vi "Read.ProcessData.ChangeIndexes.vi"(4 "length":i32=-1, 6 "index":i32, 8 "error in (no error)":errorcluster, 10 "timeout ms":i32, 11 "Read in":refnum<class "Read.lvclass">) -> (0 "error out":errorcluster, 1 "Timeout?":bool, 2 "Data":dbl[](array[numeric]), 3 "Read out":refnum<class "Read.lvclass">, 5 "change idexes":i32[](array[numeric]))   [LabVIEW 2015, in "Data Access Engine.lvlib" / "Read.lvclass"]
uses:
  Read.lvclass
  Read.lvclass/Read.ctl
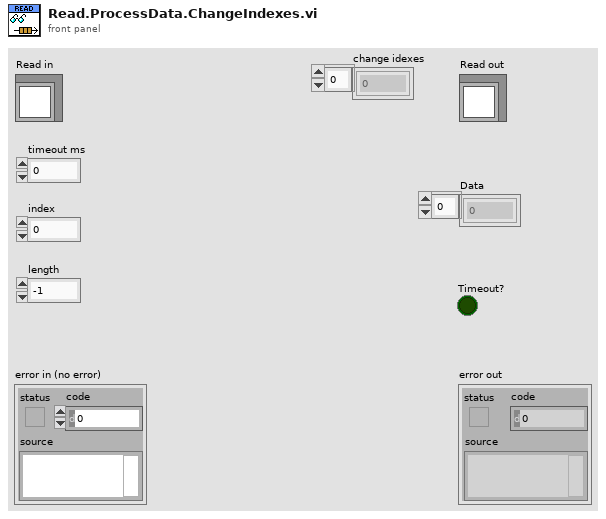
[diagram p1: front panel]
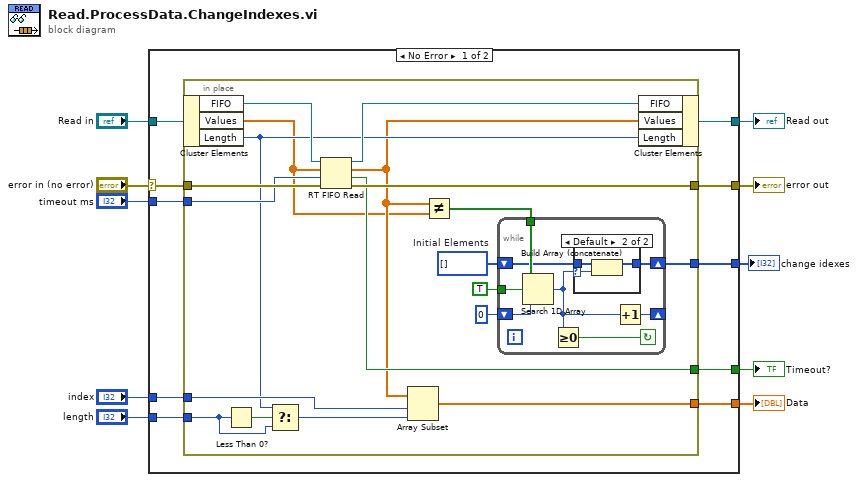
[diagram p0: block diagram]
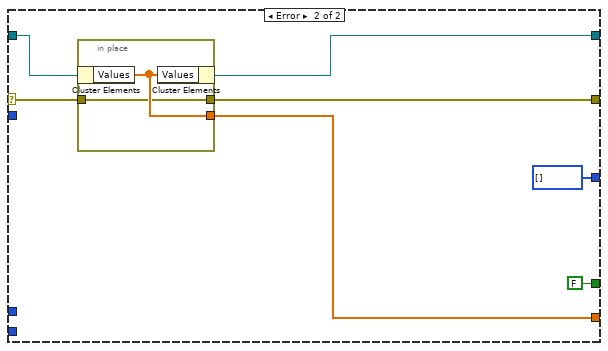
[diagram p3: hidden frame]
diagram:
  n1 = case shown="No Error" "error in (no error)" {
    selector: "error in (no error)" -> [w18 w57]
    tunnel: [w17 w53] -> w9
    tunnel: [w19 w55] -> w7
    tunnel: "Read in" -> [w20 w56]
    tunnel: "timeout ms" -> [w16 _]
    tunnel: [w15 w54] -> w5
    tunnel: [w14 FALSE ("empty?")] -> w4
    tunnel: "length" -> [w13 _]
    tunnel: "index" -> [w12 _]
    tunnel: [w11 i32[] [] ("Initial Elements")] -> w1
    frame No Error {
      n2 = in-place {
        in-place-border: w18 -> [w37]
        in-place-border: [w36] -> w17
        in-place-border: w16 -> [w35]
        in-place-border: [w29] -> w15
        in-place-border: [w34] -> w14
        in-place-border: w13 -> [w32]
        in-place-border: w12 -> [w30]
        in-place-border: [w21] -> w11
        w26 = i32[] []  # Initial Elements
        n3 = in-place-cluster #1(w20) -> ("FIFO"=w39:refnum<k33>, "Values"=w23:dbl[], "Length"=w28:i32)
        n4 = Less Than 0?(x=w32) -> (x < 0?=w33:bool)
        n5 = Select(t=w28, s=w33, f=w32) -> (s? t:f=w31:i32)
        n6 = RT FIFO Read(0:w39, 1:w23, 2:w35, 3:w37) -> (8:w38:refnum<k33>, 9:w24:dbl[], 10:w34:bool, 11:w36:errorcluster)  [unwired: 1 out]
        n7 = Array Subset(array=w24, index=w30, length=w31) -> (w29:dbl[])
        n8 = Not Equal?(x=w24, y=w23) -> (x != y?=w22:bool[])
        n9 = while {
          shift-right: [w40] -> _
          shift-left: 0 ("Start Index (0)") -> [w47]
          shift-right: [w44] -> w21
          shift-left: w26 -> [w45]
          tunnel: w22 -> [w46]
          tunnel: TRUE -> [w43]
          stop <- w41 continue-if-true
          n10 = Search 1D Array(1D array=w46, element=w43, start index (0)=w47) -> (index of element=w42:i32)
          n11 = Greater Or Equal To 0?(x=w42) -> (x >= 0?=w41:bool)
          n12 = case shown="Default" w42 {
            selector: w42 -> [_ w51]
            tunnel: w45 -> [w48 w50]
            tunnel: [w48 w49] -> w44
            frame -1 {
            }
            frame Default {
              n13 = Build Array (concatenate)(w50, w51) -> (w49:i32[])
            }
          }
          n14 = Increment(x=w42) -> (x+1=w40:i32)
        }
        n15 = in-place-cluster #1("FIFO"=w38, "Values"=w24, "Length"=w28) -> (w19:refnum<class "Read.lvclass">)
      }
    }
    frame Error {
      n16 = in-place {
        in-place-border: w57 -> [w59]
        in-place-border: [w59] -> w53
        in-place-border: [w60] -> w54
        n17 = in-place-cluster #2(w56) -> ("Values"=w60:dbl[])
        n18 = in-place-cluster #2("Values"=w60) -> (w55:refnum<class "Read.lvclass">)
      }
    }
  }
  "error out" <- w9
  "Read out" <- w7
  "Data" <- w5
  "Timeout?" <- w4
  "change idexes" <- w1
